vi "Rampe e compensazioni V F C.vi"(0 "Stato Rampe":refnum<vi>, 1 "Parametri inv freno":refnum<vi>, 2 "lingua":refnum<vi>, 3 "RPM PROVA":refnum<vi>, 5 "stato Parametri rampe e comp":refnum<vi>, 7 "COPPIA DI FRENATURA [Nm]":refnum<vi>, 9 "Tipo alimentatore DC":refnum<vi>, 11 "V F Prova":refnum<vi>, 12 "Tipo motore":refnum<vi>, 13 "Stato strumenti":refnum<vi>, 14 "Forza controllo vel":refnum<vi>) -> (15 "error out":errorcluster)   [LabVIEW 2019]
uses:
  Parametri rampe e comp.ctl
  <vilib>/ptbypt/NI_PtbyPt.lvlib
  PROVE/tensione simulata.vi
  cDAQ_PLC Folder/cDAQ/AO List.ctl
  cDAQ_PLC Folder/cDAQ/SET SINGLE AO.ctl
  Global_tutti_iDati.vi
  Global_scelta_banco.vi
  Global Modulo lingua.vi
  Global Coppia max tors.vi
panel:
  in  "exit":bool
  out "Stato Rampe":T1 {"Rampa C" scale=0.0..500.0; "Rampa V" scale=0.0..400.0; "Rampa Hz" scale=0.0..50.0}
  in  "precisione kw":dbl
  in  "RPM":dbl
  in  "RPM nom":dbl
  in  "P resa letta":dbl
  in  "P imp":dbl
  out "tensione stabilizzata":bool
  out "coppia stabilizzata":bool caption="Grandezza stabilizz?"
  out "Stato":string
  in  "set V (V)":dbl
  out "stato Parametri rampe e comp":T2={"Frequenza"={"Tempo rampa (s)"=0.0, "Tempo stabiliz (s)"=0.0}, "Tensione"={"Tempo rampa (s)"=0.0, "Tempo stabiliz rampa(s)"=0.0, "Compensaz attiva?"=TRUE, "Precisione"=1.0, "Delta compensazione max"=30.0, "Time attesa stabiliz comp (s)"=5.0}, "Coppia"={"Tempo rampa (s)"=0.0, "Tempo stabiliz rampa(s)"=0.0, "Compensaz attiva?"=TRUE, "Precisione"=1.0, "Delta compensazione max"=30.0, "Time attesa stabiliz comp (s)"=5.0}}
  in  "Parametri rampe e comp":T2={"Frequenza"={"Tempo rampa (s)"=0.0, "Tempo stabiliz (s)"=0.0}, "Tensione"={"Tempo rampa (s)"=0.0, "Tempo stabiliz rampa(s)"=0.0, "Compensaz attiva?"=TRUE, "Precisione"=1.0, "Delta compensazione max"=30.0, "Time attesa stabiliz comp (s)"=5.0}, "Coppia"={"Tempo rampa (s)"=0.0, "Tempo stabiliz rampa(s)"=0.0, "Compensaz attiva?"=TRUE, "Precisione"=1.0, "Delta compensazione max"=30.0, "Time attesa stabiliz comp (s)"=5.0}}
  out "Coppia letta":dbl
  out "Tensione letta":dbl
  out "fine rampa C":bool
  in  "set (C)":dbl
  out "OUT C":dbl
  out "fine rampa V":bool
  out "OUT V":dbl
  out "OUT HZ":dbl
  in  "set (Hz)":dbl
  out "fine rampa HZ":bool
  # "controlli per simulazione"
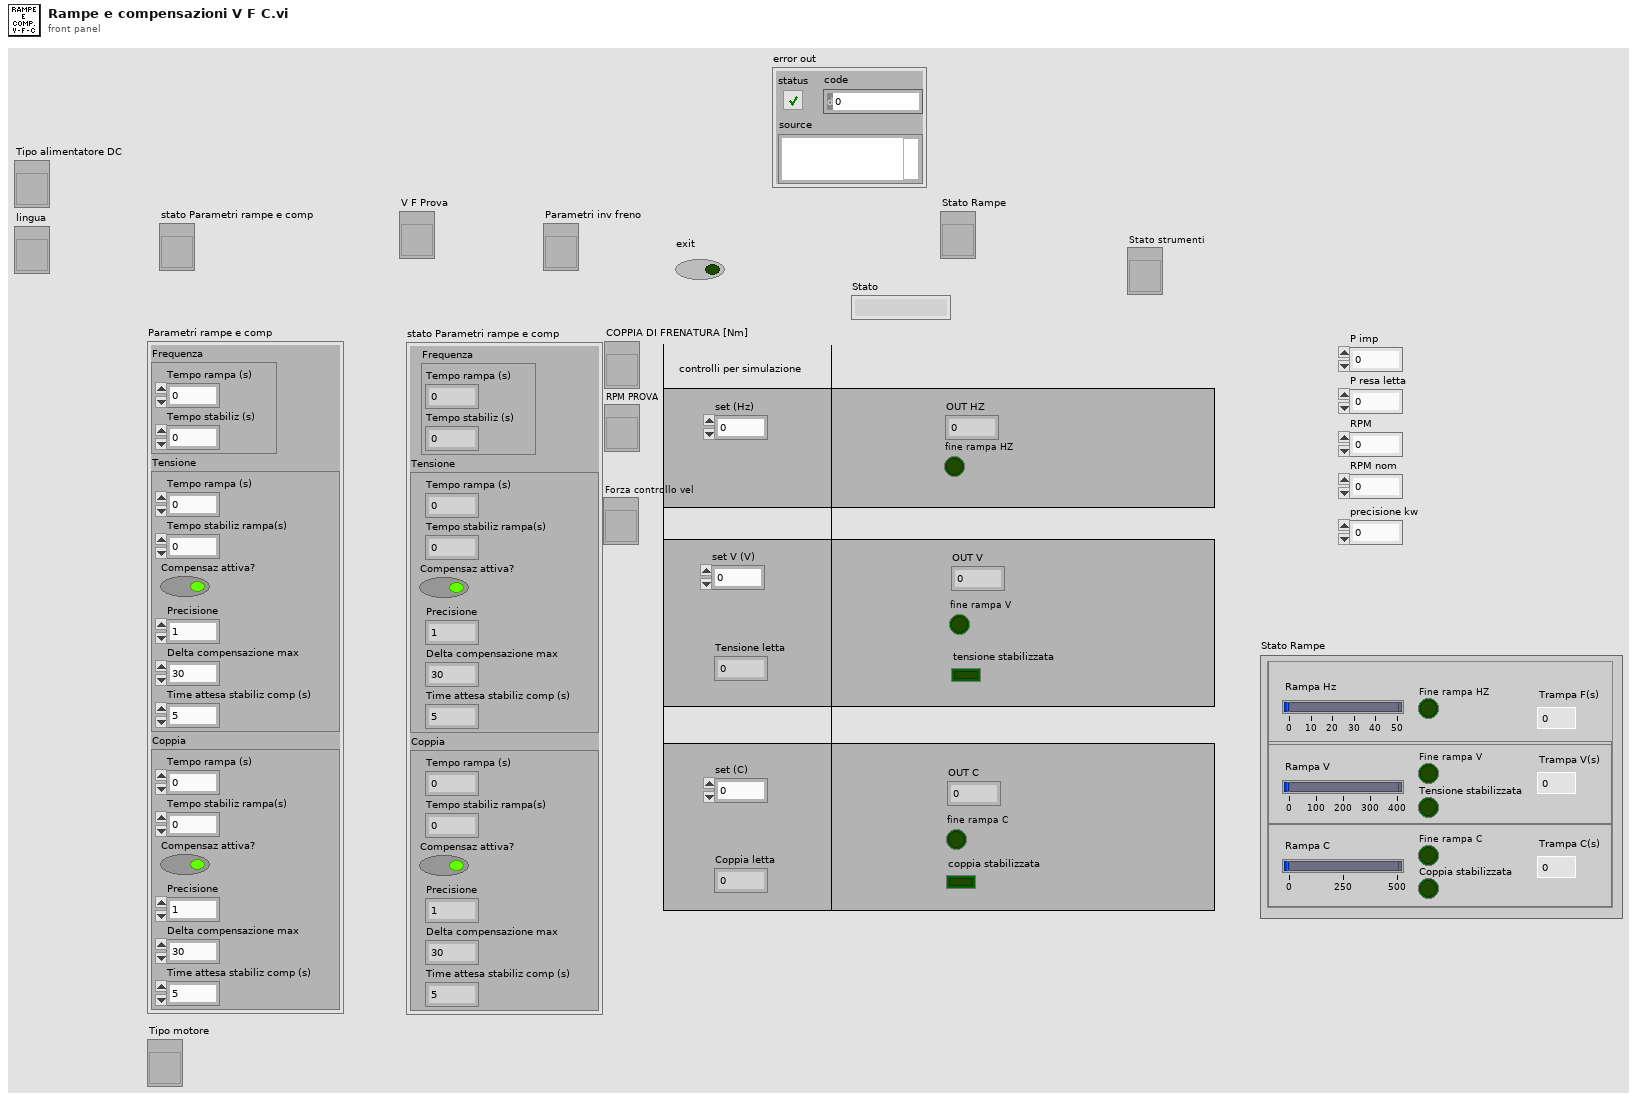
[diagram p1: front panel]
types:
  T1 = cluster{"Fine rampa HZ":bool, "Fine rampa V":bool, "Tensione stabilizzata":bool, "Fine rampa C":bool, "Coppia stabilizzata":bool, "Rampa Hz":dbl, "Rampa V":dbl, "Rampa C":dbl, "Trampa F(s)":dbl, "Trampa V(s)":dbl, "Trampa C(s)":dbl}
  T2 = typedef "Parametri rampe e comp.ctl" = cluster{"Frequenza":cluster{"Tempo rampa (s)":dbl, "Tempo stabiliz (s)":dbl}, "Tensione":cluster{"Tempo rampa (s)":dbl, "Tempo stabiliz rampa(s)":dbl, "Compensaz attiva?":bool, "Precisione":dbl, "Delta compensazione max":dbl, "Time attesa stabiliz comp (s)":dbl}, "Coppia":cluster{"Tempo rampa (s)":dbl, "Tempo stabiliz rampa(s)":dbl, "Compensaz attiva?":bool, "Precisione":dbl, "Delta compensazione max":dbl, "Time attesa stabiliz comp (s)":dbl}}
  T3 = cluster{"Message":string, "Message Data":variant}
  T4 = cluster{"name (unnamed)":string, "variant":variant}
  T5 = typedef "SET SINGLE AO.ctl" = cluster{"AO":T6, "Value":dbl}
  T6 = typedef "AO List.ctl" = enum16{"OFF: ALL AO", "Vout Variac", "Vout Freq", "Vout 3", "Vout 4", "Forza AO", "*V eccitazion", "*I eccitazione", "*Rif vel inv freno", "*Rif coppia inv freno", "Exit"}
  T7 = cluster{"WT330":bool, "CDAQ":bool, "RESIS. METER":bool, "PLC":bool, "AFE ENERGY":bool, "INV FRENO":bool, "RESISTOMAT":bool}
  T8 = typedef "Tutti_i_dati.ctl" = cluster{"Letture":T9, "Misure Wt330":cluster{"CANALE 1":cluster{"U":dbl, "I":dbl, "P":dbl, "S":dbl, "Q":dbl, "LAMB":dbl, "PHI":dbl, "FU":dbl, "FI":dbl, "NONE":dbl}, "CANALE 2":cluster{"U":dbl, "I":dbl, "P":dbl, "S":dbl, "Q":dbl, "LAMB":dbl, "PHI":dbl, "FU":dbl, "FI":dbl, "NONE":dbl}, "CANALE 3":cluster{"U":dbl, "I":dbl, "P":dbl, "S":dbl, "Q":dbl, "LAMB":dbl, "PHI":dbl, "FU":dbl, "FI":dbl, "NONE":dbl}, "SIGMA":cluster{"U":dbl, "I":dbl, "P":dbl, "S":dbl, "Q":dbl, "LAMB":dbl, "PHI":dbl, "FU":dbl, "FI":dbl, "NONE":dbl}}, "statoAO_PLC":T10, "statoDO_cDaq":T11, "StatoDO_PLC":T12, "statoAO_Cdaq":T13}
  T9 = typedef "LettureCDAQ_PLC.ctl" = cluster{"DI-logici":cluster{"Sistema OK":bool, "Inverter mot freno Run":bool, "Collaudo abilitato":bool, "Potenza trifase abilitata":bool, "Potenza monofase abilitata":bool, "Potenza DC abilitata":bool, "Potenza DC MP abilitata":bool, "Potenza DC abilitata no WT":bool, "Potenza DC MP abilitata no WT":bool, "Potenza Eccitazione abilitata":bool, "Start alimentazione AC":bool, "Start alimentazione DC":bool, "Start eccitazione DC":bool, "Controllo coppia abilitato":bool, "Senso rotazione motore freno":bool, "Teler ramo WT abilitato":bool, "Teler princ Resist abilitato":bool, "Teler corto fasi":bool, "Ramo 1 resistomat":bool, "Ramo 2 resistomat":bool, "Ramo 3 resistomat":bool, "Stop prova":bool, "Reset allarme":bool, "Rot bloccato (0= bloccato)":bool, "Scala torsiometro":bool}, "Termocoppie":cluster{"Tamb (°C)":dbl, "TC 2":dbl, "TC 3":dbl, "TC 4":dbl}, "AI cDAQ":cluster{"C[Nm] 1":dbl, "C[Nm] 2":dbl}, "Counters":cluster{"RPM 1":dbl, "RPM 2":dbl}, "Stato DI_Cdaq":cluster{"Motore monofase abil":bool, "Motore trifase abil":bool, "Uscita generale abil":bool, "2nd ch res meter abil":bool, "TA selezionati":bool, "Pulsante Start prova":bool, "Pulsante Stop prova":bool, "Pulsante Reset allarmi":bool, "Secondari TA aperti":bool, "Res meter abil":bool, "Scorta 1":bool, "Scorta 2":bool, "Scorta 3":bool, "Scorta 4":bool, "Scorta 5":bool, "Scorta 6":bool, "Scorta 7":bool, "Scorta 8":bool, "Scorta 9":bool, "Scorta 10":bool, "Scorta 11":bool, "Scorta 12":bool, "Scorta 13":bool, "Scorta 14":bool, "Scorta 15":bool, "Scorta 16":bool, "Scorta 17":bool, "Scorta 18":bool, "Scorta 19":bool, "Scorta 20":bool, "Scorta 21":bool, "Scorta 22":bool}, "Stato DI_PLC":cluster{"Diff Relay On":bool, "Em Stop Mod ok":bool, "Secur Bar Mod ok":bool, "Int PwPan Fan enab":bool, "Start Test P-b":bool, "Stop Test P-b":bool, "Reset Alarms P-b":bool, "Single-ph M enab":bool, "Three-ph M enab":bool, "Gen Output enab":bool, "Inv  11kW enab":bool, "Inv 3kW enab":bool, "AFE enab":bool, "P.S. Brushless M enab":bool, "Brush M started (scorta)":bool, "M Tested Sig enab":bool, "Br M 4kW Fan enab":bool, "Blocked Rot 1":bool, "Blocked Rot 2":bool, "Klixon Br Res 1":bool, "Klixon Br Res 2":bool, "Klixon Line Reac":bool, "Klixon S.L. Reac":bool, "Res Meter enab":bool, "2Ch Res Meter enab":bool, "Bypass Res Meter":bool, "TA selected":bool, "TA bypassed":bool, "Direct Line sel":bool, "Branch WT enab":bool, "Branch 1 Resist":bool, "Branch 2 Resist":bool, "Branch 3 Resist":bool, "Short Circ windings":bool, "Sec1 coil sel":bool, "Sec2 Coil sel":bool, "Inv 11kW ready":bool, "Inv 3kW ready":bool, "AFE ready":bool, "P.S. Direct Line enab":bool, "Scorta 1":bool, "Scorta 2":bool, "Scorta 3":bool, "Scorta 4":bool, "Scorta 5":bool, "Scorta 6":bool, "*Inv 11kW started":bool, "*Inv 3kW started":bool, "*AFE started":bool, "*Bench 300W":bool, "*Bench 3kW":bool}, "Letture res meter":cluster{"Res Ch1":dbl, "Res Ch2":dbl}, "Banco selez":cluster{"C[Nm]":dbl, "RPM":dbl}, "AI plc":cluster{"Allarmi_1":dbl, "Allarmi_2":dbl, "RPM inv 3kW":dbl, "RPM inv 11kW":dbl}, "Letture resistomat":cluster{"Res Ch1":dbl, "Res Ch2":dbl}}
  T10 = typedef "statoAO_plc.ctl" = cluster{"Rif vel freno":dbl, "Rif coppia freno":dbl, "Rif tens AFE":dbl, "Rif freq AFE":dbl}
  T11 = typedef "statoDO.ctl" = cluster{"Abilita motore monofase":bool, "Abilita motore trifase":bool, "Abilita uscita generale":bool, "Abilita res meter":bool, "Abilita 2nd canale res meter":bool, "Bypass res meter":bool, "Ctrl torsiometro 1":bool, "Scala torsiometro 1":bool, "Ctrl torsiometro 2":bool, "Scala torsiometro 2":bool, "Seleziona TA":bool, "Seleziona linea diretta":bool, "Seleziona spire TA":bool, "Bypass TA":bool, "Lampada Test in progress":bool, "Lampada allarme":bool, "Apri TA secondari":bool, "Scorta 1":bool, "Scorta 2":bool, "Scorta 3":bool, "Scorta 4":bool, "Scorta 5":bool, "Scorta 6":bool, "Scorta 7":bool, "Scorta 8":bool, "Scorta 9":bool, "Scorta 10":bool, "Scorta 11":bool, "Scorta 12":bool, "Scorta 13":bool, "Scorta 14":bool, "Scorta 15":bool}
  T12 = typedef "StatoDO_PLC.ctl" = cluster{"Enab Single-ph M":bool, "Enab Three-ph M":bool, "Enab Gen Output":bool, "Enab Electric Lock":bool, "Reset Diff Relay":bool, "Test in Progress Lamp":bool, "Alarm Lamp":bool, "Enab Inv 11kW":bool, "Start Inv 11kW":bool, "Scorta 1":bool, "Enab Inv 3kW":bool, "Start Inv 3kW":bool, "Enab AFE":bool, "Start AFE":bool, "Enab PS Brush M":bool, "Start Brush M (scorta)":bool, "Enab M Tested Sig":bool, "Enab Fan Brak M 4kW":bool, "Enab Res Meter":bool, "Enab 2Ch Res Meter":bool, "Bypass Res Meter":bool, "Select TA":bool, "Bypass TA":bool, "Select Direct Line":bool, "Enab Branch WT":bool, "Spire TA (scorta)":bool, "Ctrl Torq Meter 50Nm":bool, "Scale Torq Meter 50Nm ":bool, "Ctrl Torq Meter 5Nm":bool, "Scale Torq Meter 5Nm":bool, "Branch 1 resist":bool, "Branch 2 resist":bool, "Branch 3 resist":bool, "Short Circ Windings":bool, "Sel  Windings 300V":bool, "Sel  Windings 450V":bool, "P.S. Direct Line":bool, "Scorta 2":bool, "Scorta 3":bool, "Scorta 4":bool, "Scorta 5":bool, "Scorta 6":bool, "*Reset Allarmi":bool, "*Senso Rotaz freno":bool, "*Controllo Coppia":bool, "*Abilita freno":bool, "*Marcia freno":bool, "*Watch dog":bool, "*Bench 300W":bool, "*Bench 3kW":bool}
  T13 = typedef "StatoAO_cdaq.ctl" = cluster{"Vout variac":dbl, "AO 2":dbl, "AO 3":dbl, "AO 4":dbl}
  T14 = cluster{"Tempo rampa (s)":dbl, "Tempo stabiliz rampa(s)":dbl, "Compensaz attiva?":bool, "Precisione":dbl, "Delta compensazione max":dbl, "Time attesa stabiliz comp (s)":dbl}
  T15 = cluster{"Tempo rampa (s)":dbl, "Tempo stabiliz (s)":dbl}
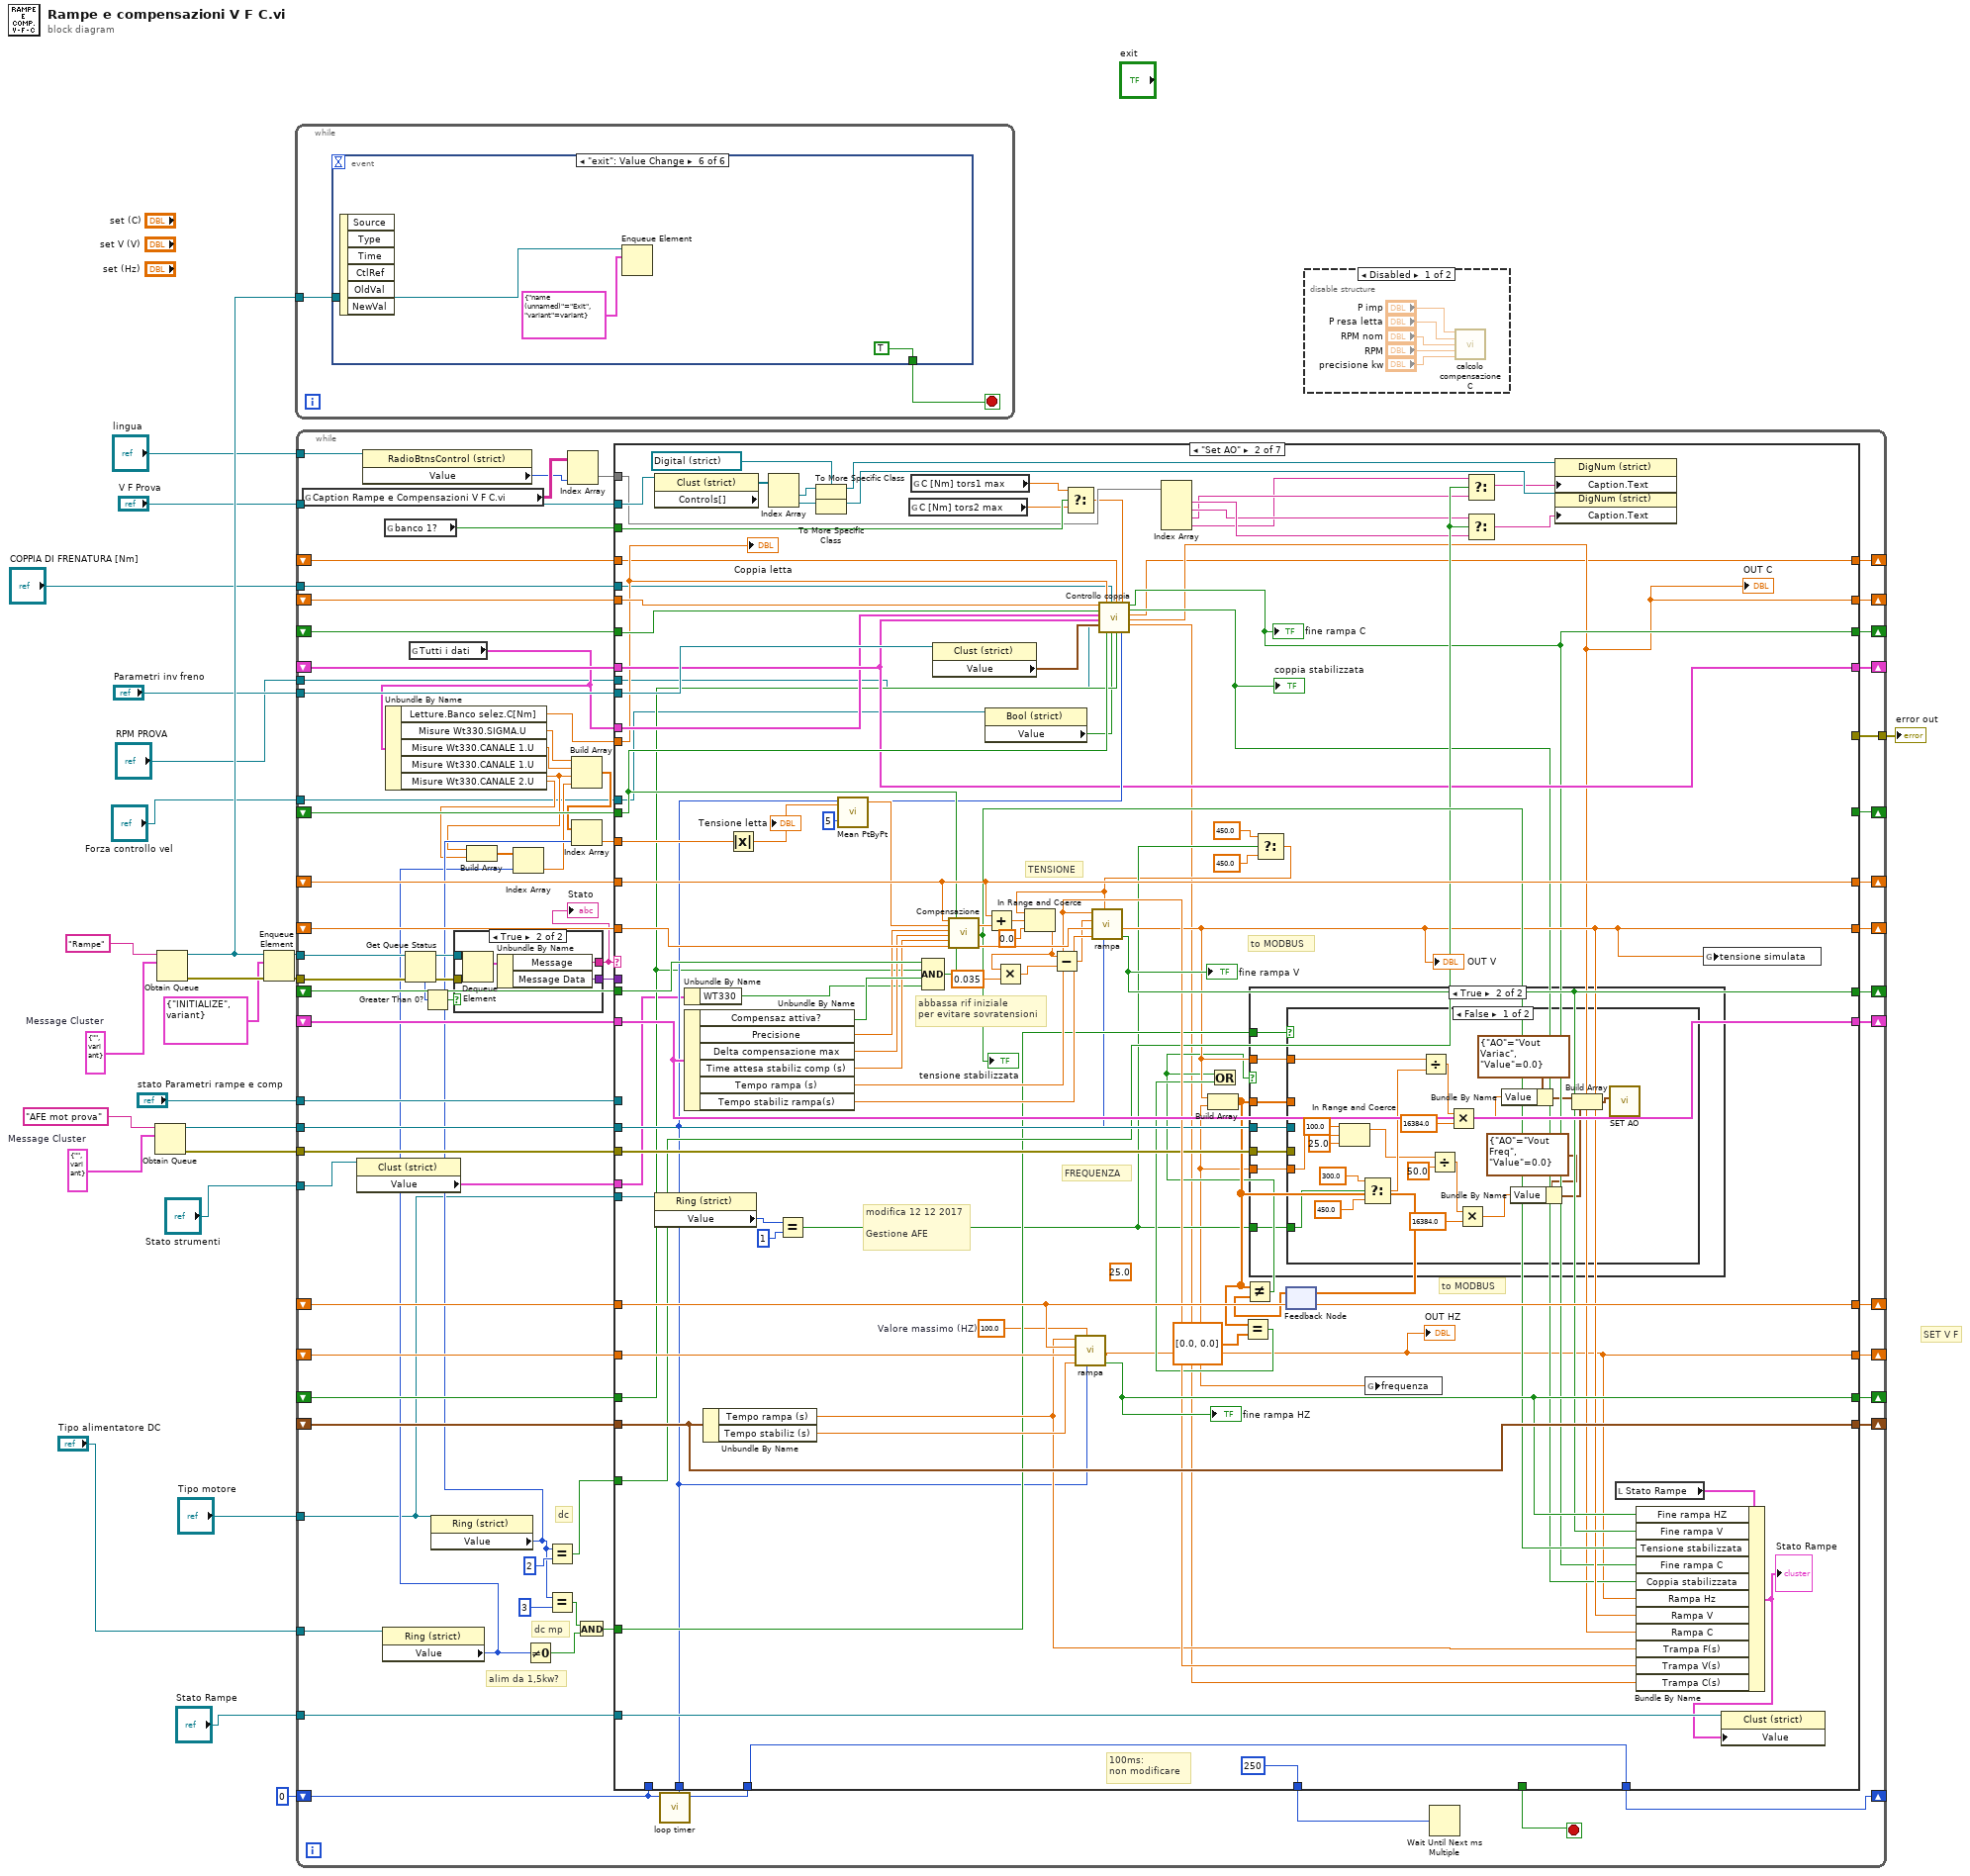
[diagram p0: block diagram]
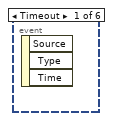
[diagram p3: hidden frame]
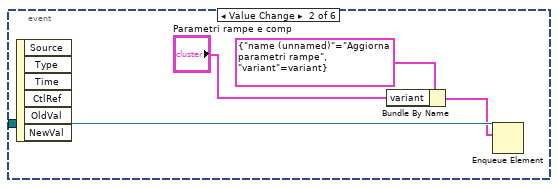
[diagram p4: hidden frame]
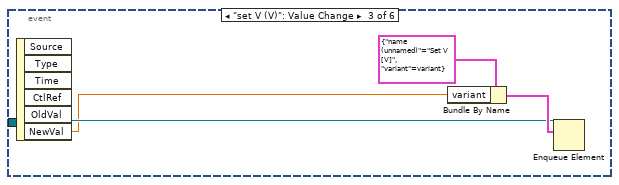
[diagram p5: hidden frame]
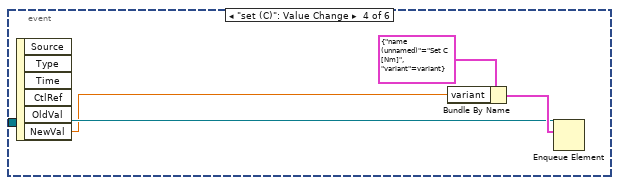
[diagram p6: hidden frame]
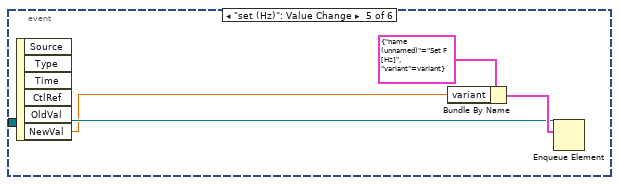
[diagram p7: hidden frame]
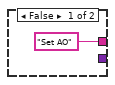
[diagram p8: hidden frame]
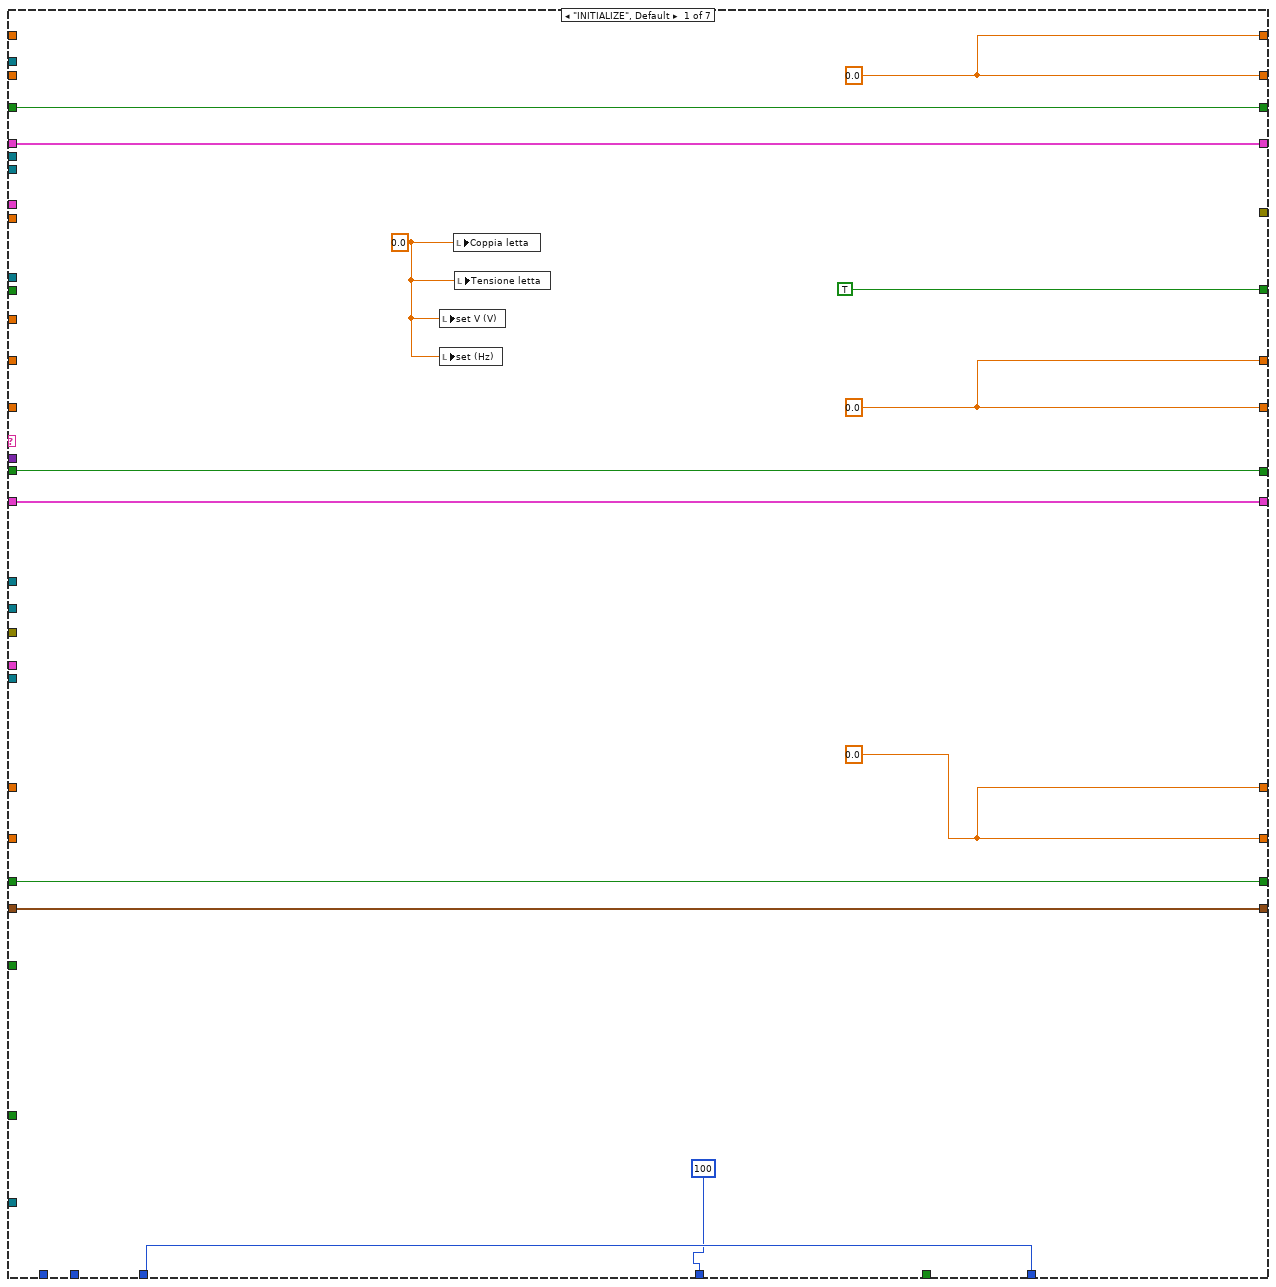
[diagram p9: hidden frame]
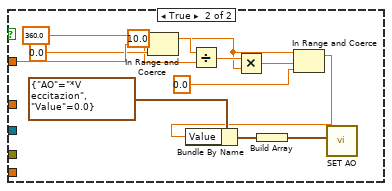
[diagram p11: hidden frame]
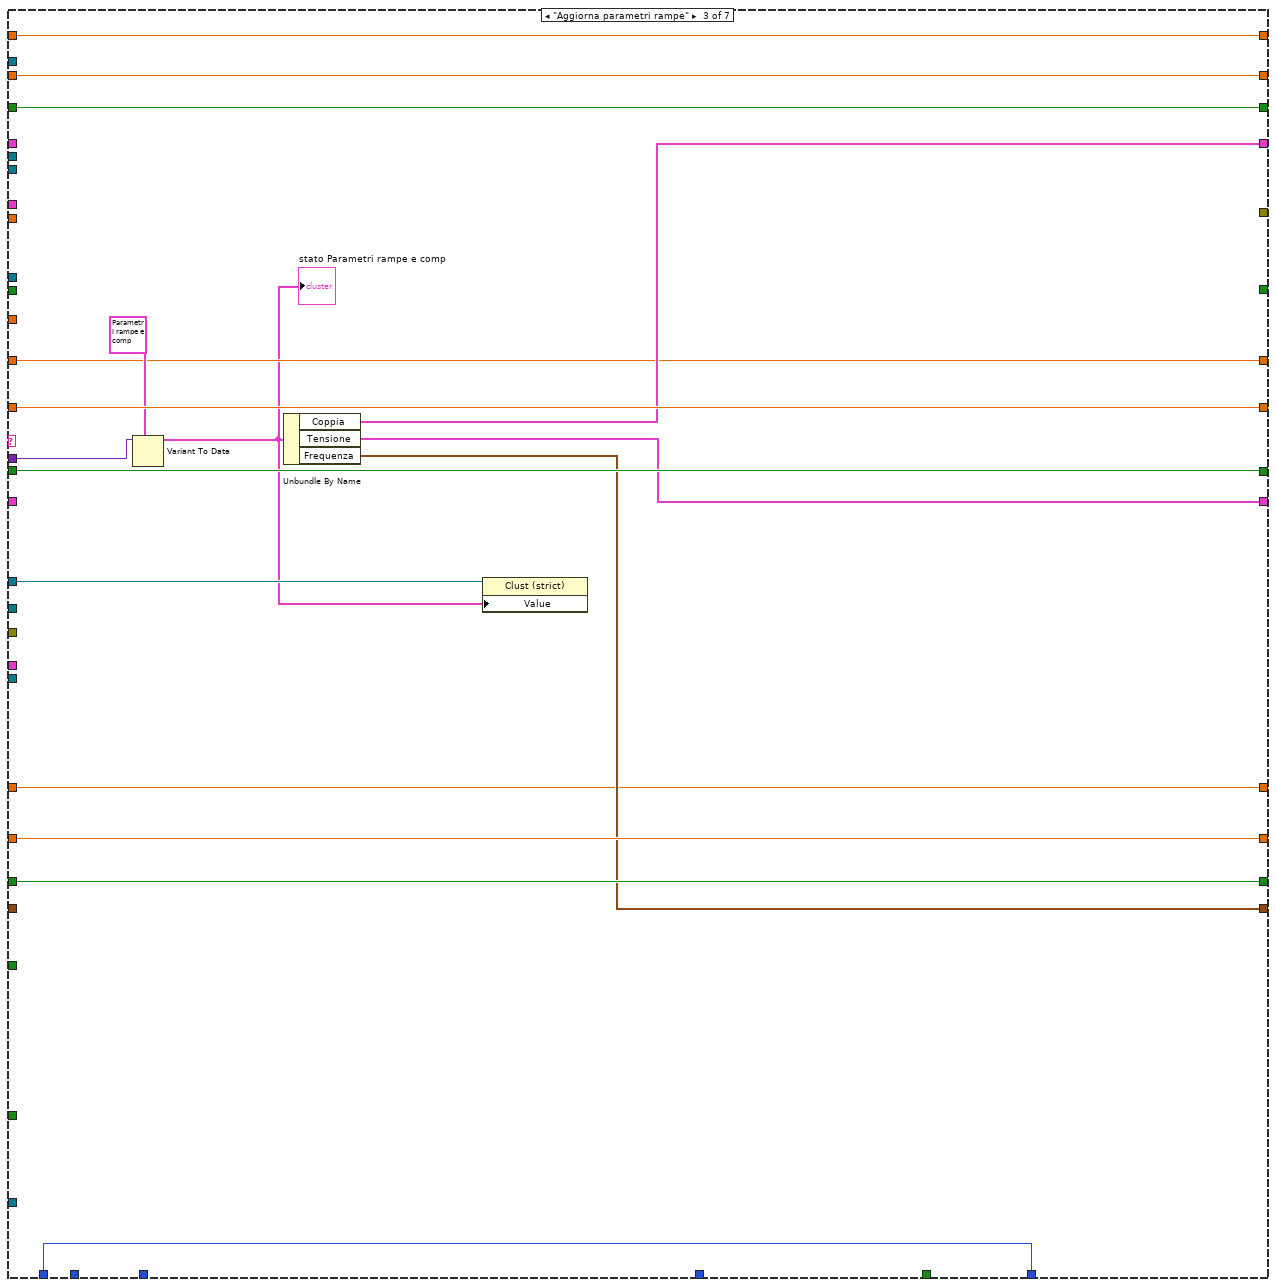
[diagram p12: hidden frame]
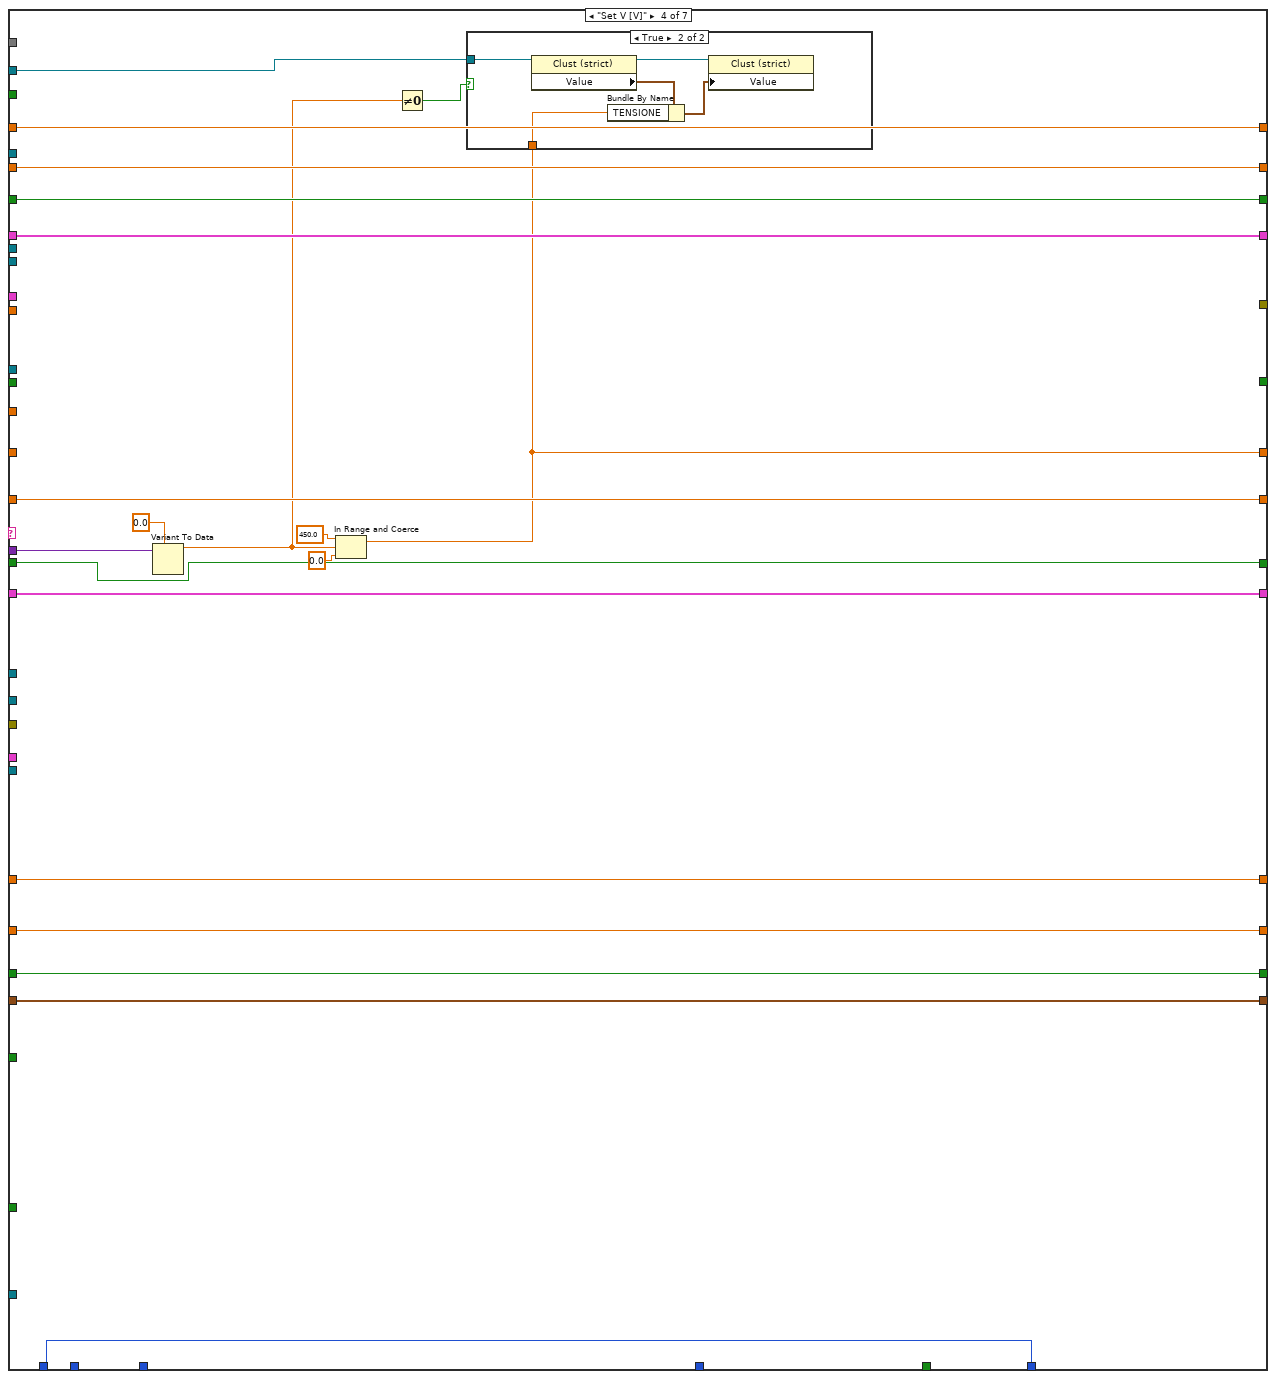
[diagram p13: hidden frame]
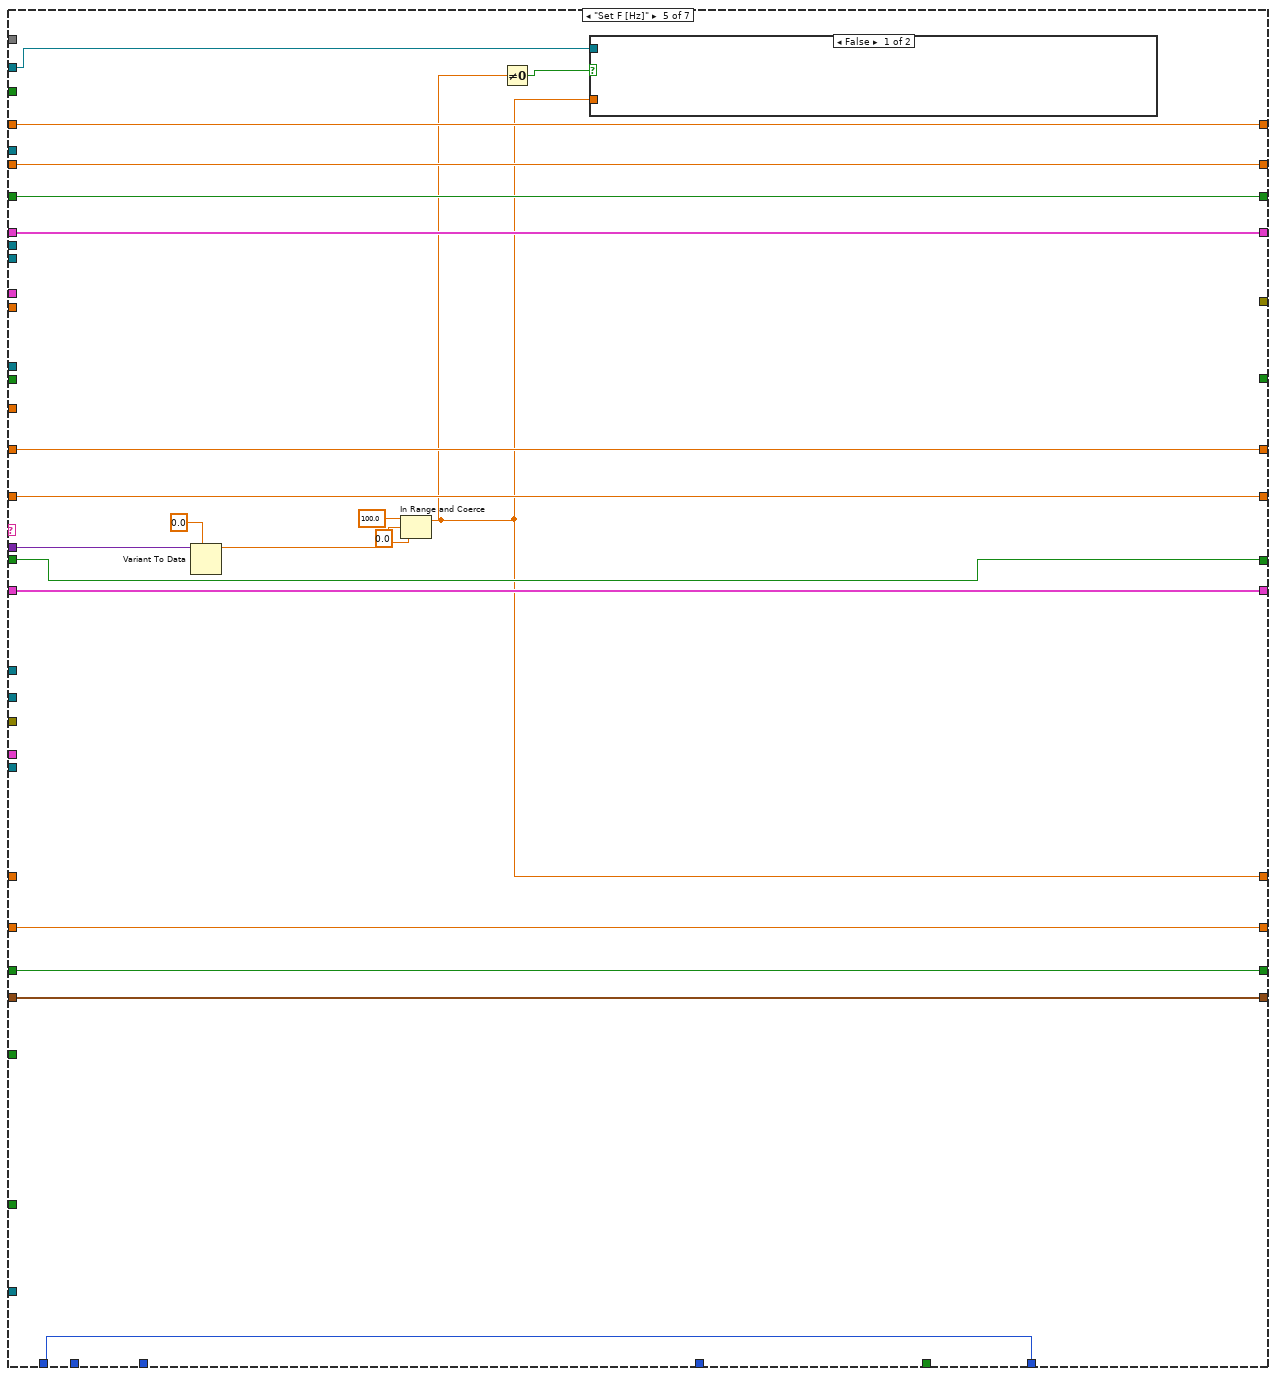
[diagram p15: hidden frame]
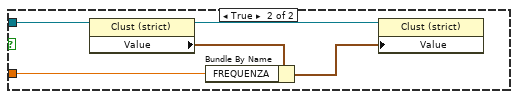
[diagram p16: hidden frame]
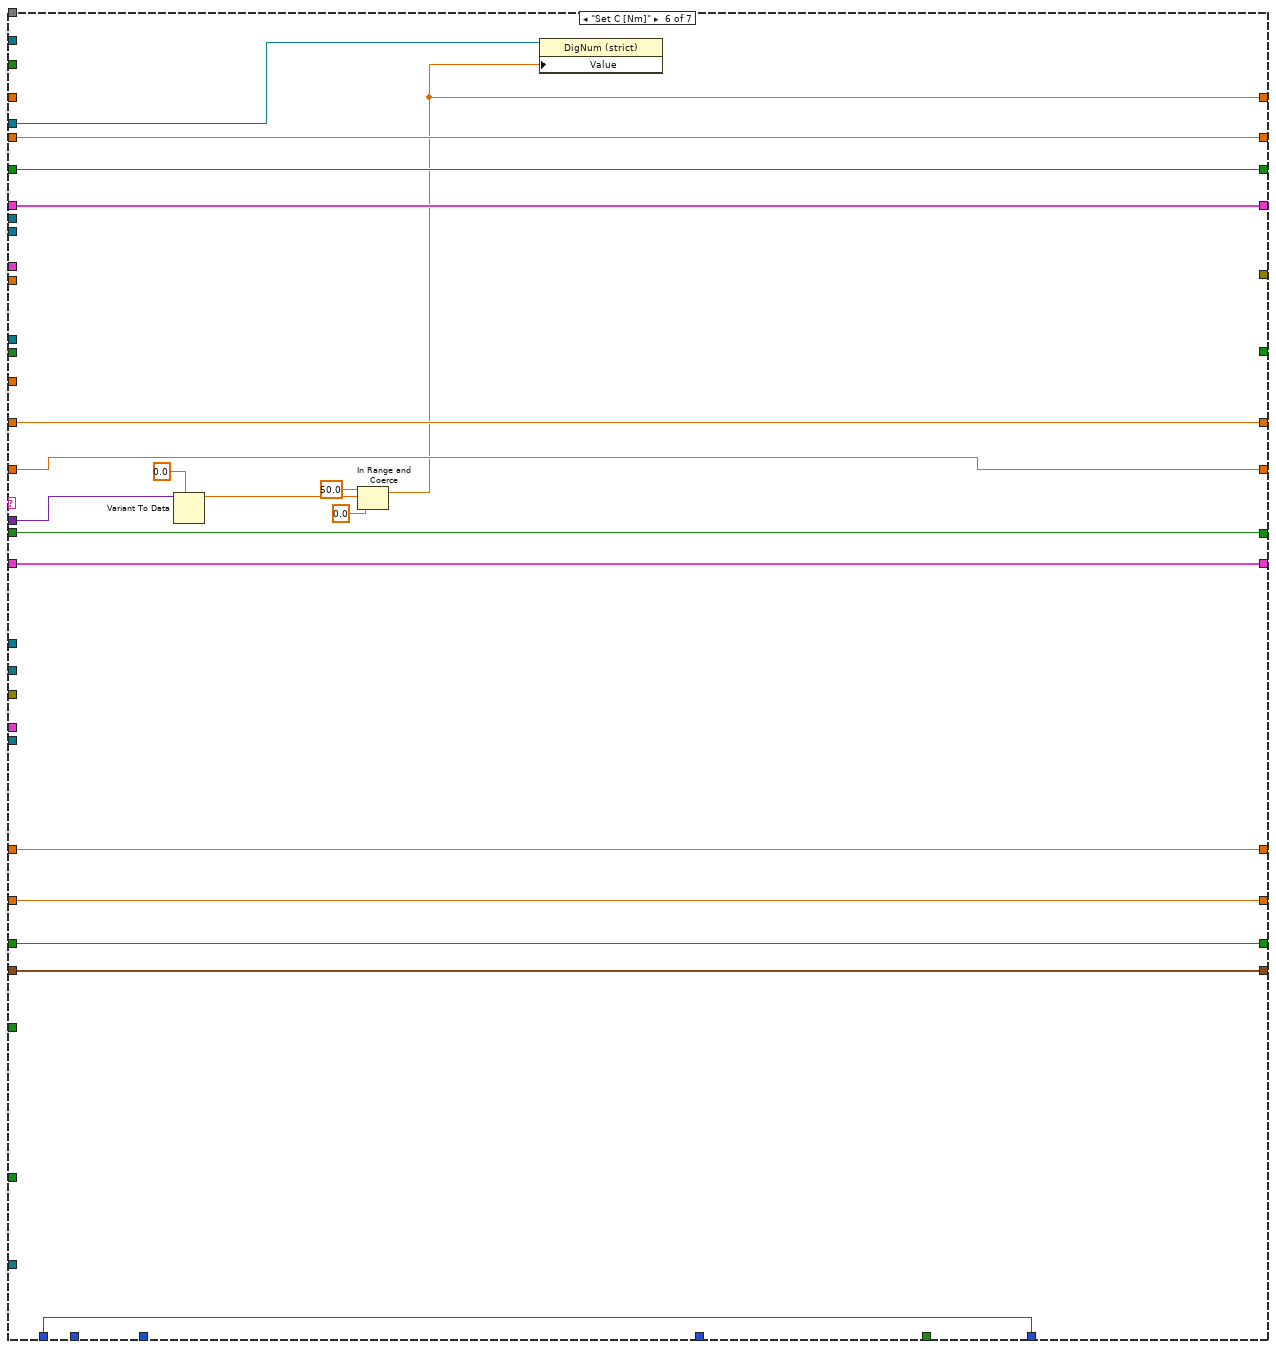
[diagram p17: hidden frame]
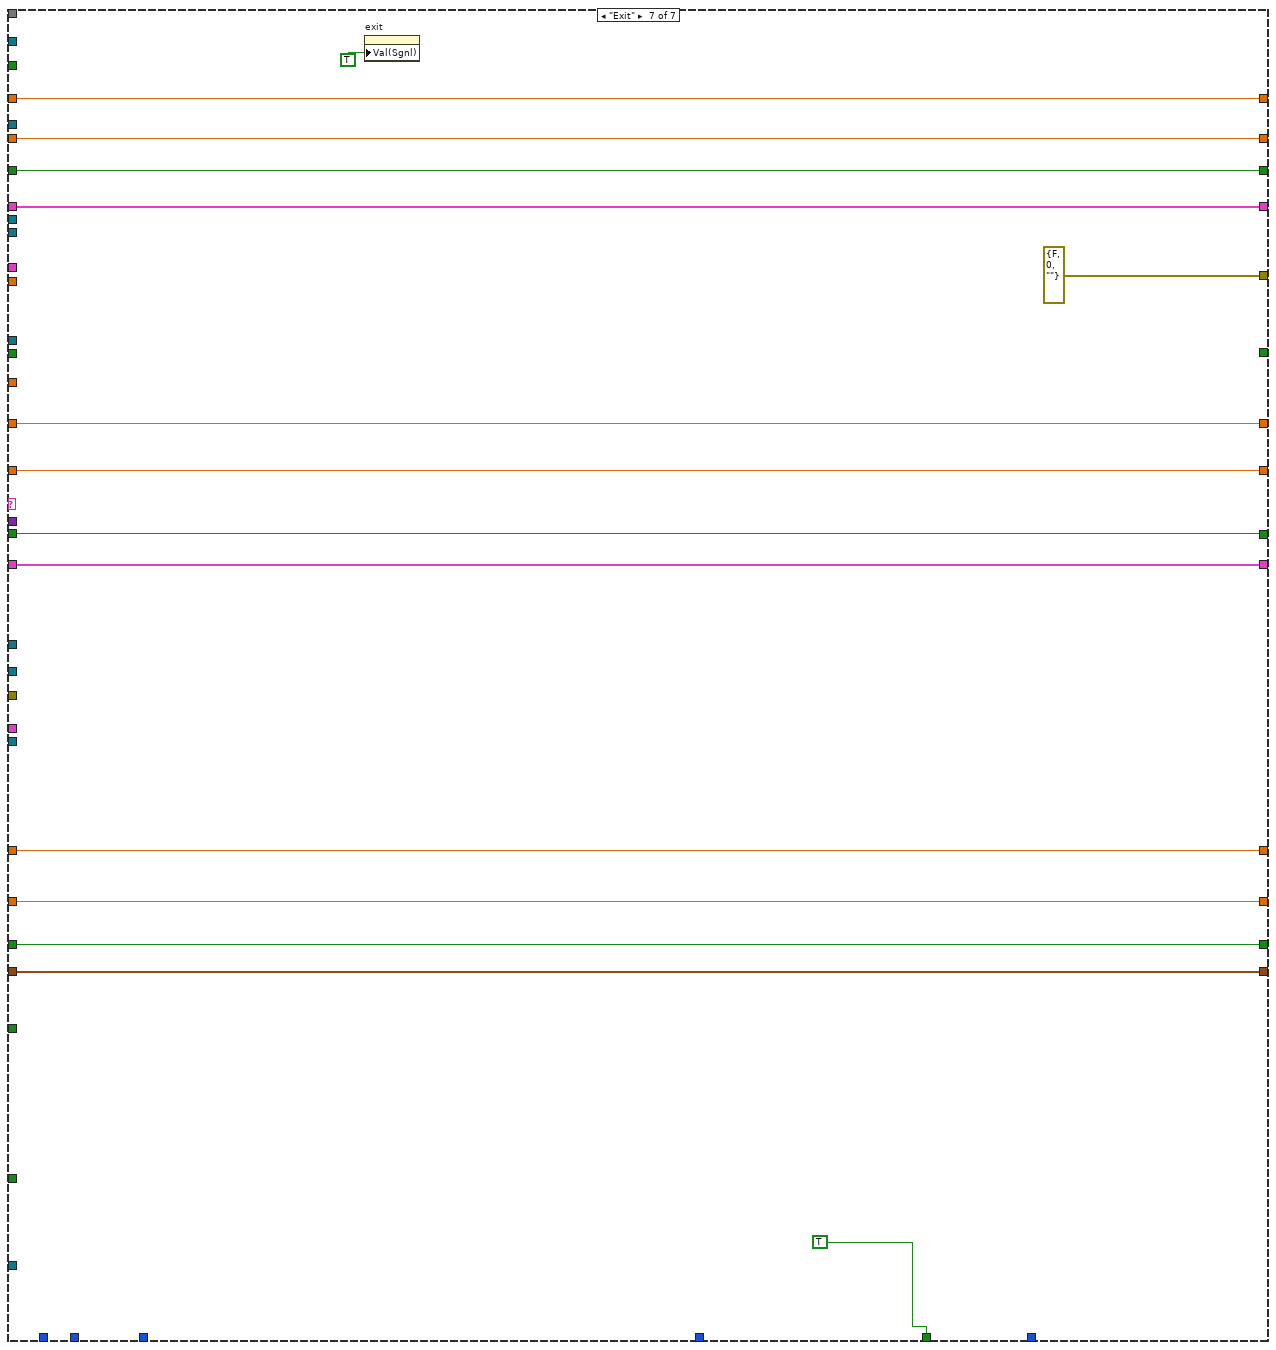
[diagram p18: hidden frame]
diagram:
  w13 = T3 {"Message"="", "Message Data"=variant}  # Message Cluster
  w17 = T3 {"Message"="", "Message Data"=variant}  # Message Cluster
  # "SET V F"
  n1 = Obtain Queue(name (unnamed)="AFE mot prova", element data type=w13) -> (queue out=w11:refnum<queue>, error out=w10:errorcluster)  [unwired: 3 in, 1 out]
  n2 = Obtain Queue(name (unnamed)="Rampe", element data type=w17) -> (queue out=w18:refnum<queue>, error out=w23:errorcluster)  [unwired: 3 in, 1 out]
  n3 = Enqueue Element(queue=w18, element=T4 {"name (unnamed)"="INITIALIZE", "variant"=variant}, error in (no error)=w23) -> (queue out=w21:refnum<queue>, error out=w22:errorcluster)  [unwired: 1 in, 1 out]
  n4 = while {
    tunnel: w18 -> [w26]
    stop <- w25 stop-if-true
    n5 = event shown="[5] \"exit\": Value Change" {
      selector: _ -> [_ _ _ _ _ _]
      dyn-events: _ -> [_ _ _ _ _ _]
      timeout: _ -> [_ _ _ _ _ _]
      tunnel: w26 -> [_ w30 w32 w36 w40 w43]
      tunnel: [_ _ _ _ _ TRUE] -> w25
      event Timeout {
        n6 = event-data() -> ()  [unwired: 1 in, 3 out]
      }
      event Value Change {
        n7 = event-data() -> ()  [unwired: 1 in, 6 out]
        n8 = Bundle By Name(cluster=T4 {"name (unnamed)"="Aggiorna parametri rampe", "variant"=variant}, "variant"="Parametri rampe e comp") -> (w29:T4)
        n9 = Enqueue Element(queue=w30, element=w29) -> ()  [unwired: 2 in, 3 out]
      }
      event "set V (V)": Value Change {
        n10 = event-data() -> ("NewVal"=w31:dbl)  [unwired: 1 in, 5 out]
        n11 = Bundle By Name(cluster=T4 {"name (unnamed)"="Set V [V]", "variant"=variant}, "variant"=w31) -> (w34:T4)
        n12 = Enqueue Element(queue=w32, element=w34) -> ()  [unwired: 2 in, 3 out]
      }
      event "set (C)": Value Change {
        n13 = event-data() -> ("NewVal"=w35:dbl)  [unwired: 1 in, 5 out]
        n14 = Bundle By Name(cluster=T4 {"name (unnamed)"="Set C [Nm]", "variant"=variant}, "variant"=w35) -> (w38:T4)
        n15 = Enqueue Element(queue=w36, element=w38) -> ()  [unwired: 2 in, 3 out]
      }
      event "set (Hz)": Value Change {
        n16 = event-data() -> ("NewVal"=w39:dbl)  [unwired: 1 in, 5 out]
        n17 = Bundle By Name(cluster=T4 {"name (unnamed)"="Set F [Hz]", "variant"=variant}, "variant"=w39) -> (w42:T4)
        n18 = Enqueue Element(queue=w40, element=w42) -> ()  [unwired: 2 in, 3 out]
      }
      event "exit": Value Change {
        n19 = event-data() -> ()  [unwired: 1 in, 6 out]
        n20 = Enqueue Element(queue=w43, element=T4 {"name (unnamed)"="Exit", "variant"=variant}) -> ()  [unwired: 2 in, 3 out]
      }
    }
  }
  n21 = while {
    shift-right: [w77] -> _
    shift-left: u32 0 ("millisecond timer OUT") -> [w76]
    shift-right: [w121] -> _
    shift-left: _ -> [w122]
    shift-right: [w120] -> _
    shift-left: _ -> [w112]
    shift-right: [w118] -> _
    shift-left: _ -> [w119]
    shift-right: [w116] -> _
    shift-left: _ -> [w113]
    shift-right: [w115] -> _
    shift-left: _ -> [w114]
    shift-right: [w111] -> _
    shift-left: _ -> [w110]
    tunnel: w21 -> [w108]
    tunnel: w22 -> [w109]
    shift-right: [w101] -> _
    shift-left: _ -> [w98]
    shift-right: [w100] -> _
    shift-left: _ -> [w96]
    shift-right: [w99] -> _
    shift-left: _ -> [w97]
    shift-right: [w95] -> _
    shift-left: _ -> [w94]
    shift-right: [w93] -> _
    shift-left: _ -> [w90]
    shift-right: [w92] -> _
    shift-left: _ -> [w91]
    shift-right: [w89] -> _
    shift-left: _ -> [w88]
    tunnel: "Stato Rampe" -> [w87]
    tunnel: "stato Parametri rampe e comp" -> [w86]
    tunnel: "V F Prova" -> [w85]
    tunnel: w11 -> [w83]
    tunnel: w10 -> [w82]
    tunnel: "Tipo motore" -> [w56]
    tunnel: "Parametri inv freno" -> [w75]
    tunnel: [w73] -> w7
    tunnel: "Tipo alimentatore DC" -> [w70]
    tunnel: "lingua" -> [w54]
    tunnel: "COPPIA DI FRENATURA [Nm]" -> [w50]
    tunnel: "Stato strumenti" -> [w49]
    tunnel: "RPM PROVA" -> [w47]
    tunnel: "Forza controllo vel" -> [w46]
    stop <- w74 stop-if-true
    # "alim da 1,5kw?"
    # "dc mp"
    # "dc"
    n22 = global read "Global Modulo lingua.vi" "Caption Rampe e Compensazioni V F C.vi"() -> (w53:string[][])
    n23 = property class="Clust (strict)"(reference=w49) -> ("Value"=w48:T7)  [unwired: 1 in, 2 out]
    n24 = property class="RadioBtnsControl (strict)"(reference=w54) -> ("Value"=w52:enum32{"Italiano", "English"})  [unwired: 1 in, 2 out]
    n25 = property class="Ring (strict)"(reference=w70) -> ("Value"=w58:u16)  [unwired: 1 in, 2 out]
    n26 = global read "Global_scelta_banco.vi" "banco 1?"() -> (w55:bool)
    n27 = Get Queue Status(queue=w108, error in (no error)=w109) -> (queue out=w104:refnum<queue>, error out=w105:errorcluster, # elements in queue=w107:i32)  [unwired: 1 in, 5 out]
    n28 = global read "Global_tutti_iDati.vi" "Tutti i dati"() -> (w57:T8)
    n29 = Unbundle By Name(w57) -> ("Letture.Banco selez.C[Nm]"=w84:dbl, "Misure Wt330.SIGMA.U"=w67:dbl, "Misure Wt330.CANALE 1.U"=w66:dbl, "Misure Wt330.CANALE 1.U"=w62:dbl, "Misure Wt330.CANALE 2.U"=w61:dbl)
    n30 = Greater Than 0?(x=w107) -> (x > 0?=w106:bool)
    n31 = property class="Ring (strict)"(reference=w56) -> ("Value"=w64:u16)  [unwired: 1 in, 2 out]
    n32 = case shown="True" w106 {
      tunnel: w105 -> [_ w128]
      tunnel: w104 -> [_ w127]
      tunnel: ["Set AO" ("Stato") w125] -> w103
      tunnel: [_ w124] -> w102
      frame False {
      }
      frame True {
        n33 = Dequeue Element(queue=w127, error in (no error)=w128) -> (element=w126:T3)  [unwired: 1 in, 3 out]
        n34 = Unbundle By Name(w126) -> ("Message"=w125:string, "Message Data"=w124:variant)
      }
    }
    "Stato" <- w103
    n35 = Build Array(w62, w61) -> (w60:dbl[])
    n36 = Index Array(array=w60, index=w58) -> (element=w59:dbl)
    n37 = Not Equal To 0?(x=w58) -> (x != 0?=w69:bool)
    n38 = Equal?(x=w64, y=u16 2) -> (x = y?=w80:bool)
    n39 = Equal?(x=w64, y=u16 3) -> (x = y?=w71:bool)
    n40 = Index Array(array=w53, index (col)=w52) -> (element=w51:string[])  [unwired: 1 in]
    n41 = Build Array(w67, w66, w62, w59) -> (w65:dbl[])
    n42 = Index Array(array=w65, index=w64) -> (element=w63:dbl)
    n43 = And(x=w71, y=w69) -> (x .and. y?=w68:bool)
    n44 = call <userlib>:"loop timer.vi"("millisecond timer IN"=w76) -> ("millisecond timer OUT"=w78:u32, "LOOP TIME (ms)"=w117:u32)  [unwired: 9 in]
    n45 = case shown="\"Set AO\"" w103 {
      tunnel: w122 -> [_ w236 w291 w307 w328 w355 w377]
      tunnel: [w133 w148 w291 w307 w328 w355 w377] -> w121
      tunnel: [w134 w188 w292 w303 w334 w358 w376] -> w120
      tunnel: w119 -> [_ w170 w293 w304 w329 w352 w375]
      tunnel: [w135 w162 w293 w304 w329 w352 w375] -> w118
      tunnel: w117 -> [_ w167 _ _ _ _ _]
      tunnel: [w136 w216 w289 w306 w331 w354 w374] -> w116
      tunnel: [w137 w215 w290 w309 w333 w357 w373] -> w115
      tunnel: w114 -> [w137 w235 w290 w309 w333 w357 w373]
      tunnel: w113 -> [w136 w152 w289 w306 w331 w354 w374]
      tunnel: w112 -> [_ w230 w292 w303 w334 w358 w376]
      tunnel: [w138 w164 w288 w311 w336 w360 w372] -> w111
      tunnel: w110 -> [w138 w166 w288 w311 w336 w360 w372]
      tunnel: w102 -> [_ _ w287 w313 w337 w361 _]
      tunnel: [w141 w165 w285 w310 w335 w359 w371] -> w101
      tunnel: [w140 w223 w284 w308 w332 w356 w370] -> w100
      tunnel: [w139 w222 w283 w305 w330 w353 w369] -> w99
      tunnel: w98 -> [w141 w165 _ w310 w335 w359 w371]
      tunnel: w96 -> [w140 w223 _ w308 w332 w356 w370]
      tunnel: w97 -> [w139 w222 _ w305 w330 w353 w369]
      tunnel: [w134 w221 w282 w297 w327 w351 w368] -> w95
      tunnel: w94 -> [_ w221 w282 _ w327 w351 w368]
      tunnel: [w133 w220 w281 w302 w320 w350 w367] -> w93
      tunnel: [w135 w146 w280 w301 w326 w344 w366] -> w92
      tunnel: w91 -> [_ w147 w280 w301 w326 _ w366]
      tunnel: w90 -> [_ w220 w281 w302 _ w350 w367]
      tunnel: [TRUE ("fine rampa") _ _ _ _ _ _] -> w89
      tunnel: w88 -> [_ w169 _ _ _ _ _]
      tunnel: w87 -> [_ w213 _ _ _ _ _]
      tunnel: w86 -> [_ _ w279 _ _ _ _]
      tunnel: w85 -> [_ w207 _ w300 w325 _ _]
      tunnel: w84 -> [_ w157 _ _ _ _ _]
      tunnel: w83 -> [_ w209 _ _ _ _ _]
      tunnel: w82 -> [_ w208 _ _ _ _ _]
      tunnel: w80 -> [_ w198 _ _ _ _ _]
      tunnel: w57 -> [_ w160 _ _ _ _ _]
      tunnel: [u32 100 ("millisecond multiple") u32 250 ("millisecond multiple") _ _ _ _ _] -> w79
      tunnel: w78 -> [w130 w196 _ _ _ _ _]
      tunnel: [w130 w196 w277 w296 w321 w346 _] -> w77
      tunnel: w76 -> [_ _ w277 w296 w321 w346 _]
      tunnel: w75 -> [_ w195 _ _ _ _ _]
      tunnel: [_ _ _ _ _ _ TRUE ("stop")] -> w74
      tunnel: [_ _ _ _ _ _ errorcluster {"status"=FALSE, "code"=0, "source"=""} ("error out")] -> w73
      tunnel: w68 -> [_ w189 _ _ _ _ _]
      tunnel: w63 -> [_ w187 _ _ _ _ _]
      tunnel: w55 -> [_ w185 _ _ _ _ _]
      tunnel: w56 -> [_ w184 _ _ _ _ _]
      tunnel: w51 -> [_ w180 _ _ _ _ _]
      tunnel: w50 -> [_ w142 _ _ _ w345 _]
      tunnel: w48 -> [_ w151 _ _ _ _ _]
      tunnel: w47 -> [_ w145 _ _ _ _ _]
      tunnel: w46 -> [_ w144 _ _ _ _ _]
      frame "INITIALIZE", Default {
        w131 = 0.0 ("Coppia reale letta")
        w135 = 0.0 ("OUT")
        w134 = 0.0 ("OUT")
        w133 = 0.0 ("OUT")
        n46 = local write "set V (V)"(w131) -> ()
        n47 = local write "set (Hz)"(w131) -> ()
        n48 = local write "Coppia letta"(w131) -> ()
        n49 = local write "Tensione letta"(w131) -> ()
      }
      frame "Set AO" {
        (unwired) 25.0 ("lower limit")
        w203 = refnum<vi> refnum ("Coppia letta")
        w149 = 100.0  # Valore massimo (HZ)
        # "abbassa rif iniziale\nper evitare sovratensioni"
        # "modifica 12 12 2017\n\nGestione AFE"
        # "100ms:\nnon modificare"
        # "to MODBUS"
        # "to MODBUS"
        # "TENSIONE"
        # "FREQUENZA"
        n50 = property class="Clust (strict)"(reference=w207) -> ("Controls[]"=w206:refnum<vi>[])  [unwired: 1 in, 2 out]
        n51 = property class="Ring (strict)"(reference=w184) -> ("Value"=w183:u16)  [unwired: 1 in, 2 out]
        n52 = Unbundle By Name(w151) -> ("WT330"=w150:bool)
        n53 = Unbundle By Name(w223) -> ("Compensaz attiva?"=w228:bool, "Precisione"=w225:dbl, "Delta compensazione max"=w226:dbl, "Time attesa stabiliz comp (s)"=w227:dbl, "Tempo rampa (s)"=w211:dbl, "Tempo stabiliz rampa(s)"=w229:dbl)
        n54 = Unbundle By Name(w222) -> ("Tempo rampa (s)"=w210:dbl, "Tempo stabiliz (s)"=w224:dbl)
        n55 = Absolute Value(x=w187) -> (abs(x)=w190:dbl)
        "Tensione letta" <- w190
        n56 = Index Array(array=w206) -> (element #1=w205:refnum<vi>, element #2=w204:refnum<vi>)  [unwired: 2 in]
        n57 = Equal?(x=w183, y=u16 1) -> (x = y?=w181:bool)
        n58 = To More Specific Class(target class=w203, reference=w205) -> (specific class reference=w202:refnum<vi>)  [unwired: 1 in, 1 out]
        n59 = To More Specific Class(target class=w203, reference=w204) -> (specific class reference=w201:refnum<vi>)  [unwired: 1 in, 1 out]
        n60 = call <vilib>:"Mean PtByPt.vi"("x"=w190, "sample length"=5) -> ("mean"=w218:dbl)  [unwired: 2 in, 1 out]
        n61 = global read "Global Coppia max tors.vi" "C [Nm] tors2 max"() -> (w174:dbl)
        n62 = global read "Global Coppia max tors.vi" "C [Nm] tors1 max"() -> (w175:dbl)
        n63 = Compound Arithmetic op=AND(w235, w152, w228, w150) -> (w233:bool)
        n64 = property class="Clust (strict)"(reference=w195) -> ("Value"=w168:cluster{"Vel max(RPM)":dbl, "Cmax (nm)":dbl})  [unwired: 1 in, 2 out]
        n65 = call "Compensazione.vi"("Grandezza target"=w221, "Grandezza reale letta"=w218, "Precisione"=w225, "Delta compensazione max"=w226, "Time attesa stabilizzazione (s)"=w227, "Grandezza attuale in"=w230, "Reset comp?"=w169, "Compensazione abilitata"=w233) -> ("compensazione"=w232:dbl, "Grandezza stabilizz?"=w214:bool, "Grandezza attuale out"=w231:dbl)  [unwired: 9 in]
        "tensione stabilizzata" <- w214
        n66 = property class="Bool (strict)"(reference=w144) -> ("Value"=w143:bool)  [unwired: 1 in, 2 out]
        n67 = Add(x=w221, y=w232) -> (x+y=w234:dbl)
        n68 = Select(t=w175, s=w185, f=w174) -> (s? t:f=w171:dbl)
        n69 = call "rampa.vi"("tempo ciclo (ms)"=w167, "Valore massimo"=w149, "Tempo di stabilizzazione (s)"=w224, "reale"=w236, "set"=w220, "tempo rampa (s)"=w210) -> ("fine rampa"=w216:bool, "OUT"=w148:dbl)  [unwired: 4 in]
        "fine rampa HZ" <- w216
        "OUT HZ" <- w148
        n70 = call "Controllo coppia.vi"("C attuale"=w170, "fine rampa C in"=w166, "Tutti i dati"=w160, "Coppia"=w165, "Cmax RPMmax\n inverter"=w168, "RPM PROVA"=w145, "Coppia letta tors"=w157, "Reset comp"=w169, "COPPIA DI FRENATURA [Nm]"=w142, "Forza controllo vel"=w143, "Set C"=w147, "Fine rampa F"=w152, "Cmax"=w171, "LOOP TIME (ms)"=w167) -> ("fine rampa C out"=w164:bool, "C stabile"=w163:bool, "Set C out"=w146:dbl, "Out C"=w162:dbl, "Tempo rampa (s)"=w161:dbl)  [unwired: 1 in]
        "OUT C" <- w162
        "fine rampa C" <- w164
        "coppia stabilizzata" <- w163
        n71 = Index Array(array=w180) -> (element #1=w179:string, element #2=w178:string, element #3=w177:string, element #4=w176:string)  [unwired: 4 in]
        n72 = Select(t=450.0 ("y"), s=w181, f=450.0) -> (s? t:f=w172:dbl)
        n73 = In Range and Coerce(upper limit=w172, x=w234, lower limit=0.0) -> (coerced(x)=w155:dbl)  [unwired: 1 out]
        n74 = Multiply(x=w155, y=0.035) -> (x*y=w154:dbl)
        n75 = Subtract(x=w155, y=w154) -> (x-y=w156:dbl)
        n76 = call "rampa.vi"("tempo ciclo (ms)"=w167, "Valore massimo"=w172, "Tempo di stabilizzazione (s)"=w229, "reale"=w231, "set"=w156, "tempo rampa (s)"=w211) -> ("fine rampa"=w215:bool, "OUT"=w188:dbl)  [unwired: 4 in]
        "fine rampa V" <- w215
        "OUT V" <- w188
        n77 = Build Array(w188, w148) -> (w193:dbl[])
        n78 = Equal?(x=w193, y=dbl[] [0.0, 0.0]) -> (x = y?=w191:bool)
        n79 = feedback-in #1(w193) -> ()
        n80 = feedback #1() -> (w194:dbl[])  [unwired: 1 in]
        n81 = Not Equal?(x=w193, y=w194) -> (x != y?=w186:bool)
        n82 = Or(x=w186, y=w191) -> ()  [unwired: 1 out]
        n83 = case shown="True" w186 {
          tunnel: w209 -> [_ w243]
          tunnel: w208 -> [_ w242]
          tunnel: w193 -> [_ w241]
          tunnel: w189 -> [_ w240]
          tunnel: w188 -> [_ w239]
          tunnel: w148 -> [_ w238]
          tunnel: w181 -> [_ w237]
          frame False {
          }
          frame True {
            n84 = case shown="False" w240 {
              tunnel: w243 -> [_ _]
              tunnel: w242 -> [_ _]
              tunnel: w241 -> [_ _]
              tunnel: w239 -> [w258 w271]
              tunnel: w238 -> [w245 _]
              tunnel: w237 -> [w251 _]
              frame False {
                n85 = In Range and Coerce(upper limit=100.0, x=w245, lower limit=25.0) -> (coerced(x)=w244:dbl)  [unwired: 1 out]
                n86 = Select(t=300.0 ("y"), s=w251, f=450.0) -> (s? t:f=w249:dbl)
                n87 = Divide(x=w258, y=w249) -> (x/y=w261:dbl)
                n88 = Divide(x=w244, y=50.0) -> (x/y=w254:dbl)
                n89 = Multiply(x=w261, y=16384.0) -> (x*y=w259:dbl)
                n90 = Multiply(x=w254, y=16384.0) -> (x*y=w256:dbl)
                n91 = Bundle By Name(cluster=T5 {"AO"=enum."Vout Variac", "Value"=0.0} ("Cluster SET AO"), "Value"=w259) -> (w263:T5)
                n92 = Bundle By Name(cluster=T5 {"AO"=enum."Vout Freq", "Value"=0.0} ("Cluster SET AO"), "Value"=w256) -> (w253:T5)
                n93 = Build Array(w263, w253) -> (w264:T5[])
                n94 = call "SET AO.vi"("Cluster SET AO"=w264) -> ()  [unwired: 10 in, 1 out]
              }
              frame True {
                w268 = 360.0 ("upper limit")
                w266 = 10.0 ("upper limit")
                n95 = In Range and Coerce(upper limit=w268, x=w271, lower limit=0.0) -> (coerced(x)=w269:dbl)  [unwired: 1 out]
                n96 = Divide(x=w269, y=w268) -> (x/y=w267:dbl)
                n97 = Multiply(x=w267, y=w266) -> (x*y=w265:dbl)
                n98 = In Range and Coerce(upper limit=w266, x=w265, lower limit=0.0) -> (coerced(x)=w272:dbl)  [unwired: 1 out]
                n99 = Bundle By Name(cluster=T5 {"AO"=enum."*V eccitazion", "Value"=0.0} ("Cluster SET AO"), "Value"=w272) -> (w275:T5)
                n100 = Build Array(w275) -> (w276:T5[])
                n101 = call "SET AO.vi"("Cluster SET AO"=w276) -> ()  [unwired: 10 in, 1 out]
              }
            }
          }
        }
        n102 = global write "tensione simulata.vi" "frequenza"(w148) -> ()
        n103 = Select(t=w176, s=w198, f=w177) -> (s? t:f=w200:string)
        n104 = Select(t=w178, s=w198, f=w179) -> (s? t:f=w199:string)
        n105 = property class="DigNum (strict)"(reference=w202, "Caption.Text"=w200) -> ()  [unwired: 1 in, 2 out]
        n106 = property class="DigNum (strict)"(reference=w201, "Caption.Text"=w199) -> ()  [unwired: 1 in, 2 out]
        n107 = local read "Stato Rampe"() -> (w217:T1)
        n108 = Bundle By Name(cluster=w217, "Fine rampa HZ"=w216, "Fine rampa V"=w215, "Tensione stabilizzata"=w214, "Fine rampa C"=w164, "Coppia stabilizzata"=w163, "Rampa Hz"=w148, "Rampa V"=w188, "Rampa C"=w162, "Trampa F(s)"=w210, "Trampa V(s)"=w211, "Trampa C(s)"=w161) -> (w212:T1)
        "Stato Rampe" <- w212
        n109 = global write "tensione simulata.vi" "tensione simulata"(w188) -> ()
        n110 = property class="Clust (strict)"(reference=w213, "Value"=w212) -> ()  [unwired: 1 in, 2 out]
        "Coppia letta" <- w157
      }
      frame "Aggiorna parametri rampe" {
        n111 = Variant To Data(type=T2 {"Frequenza"={"Tempo rampa (s)"=0.0, "Tempo stabiliz (s)"=0.0}, "Tensione"={"Tempo rampa (s)"=0.0, "Tempo stabiliz rampa(s)"=0.0, "Compensaz attiva?"=TRUE, "Precisione"=1.0, "Delta compensazione max"=30.0, "Time attesa stabiliz comp (s)"=5.0}, "Coppia"={"Tempo rampa (s)"=0.0, "Tempo stabiliz rampa(s)"=0.0, "Compensaz attiva?"=TRUE, "Precisione"=1.0, "Delta compensazione max"=30.0, "Time attesa stabiliz comp (s)"=5.0}} ("Parametri rampe e comp"), Variant=w287) -> (data=w278:T2)  [unwired: 1 in, 1 out]
        "stato Parametri rampe e comp" <- w278
        n112 = Unbundle By Name(w278) -> ("Coppia"=w285:T14, "Tensione"=w284:T14, "Frequenza"=w283:T15)
        n113 = property class="Clust (strict)"(reference=w279, "Value"=w278) -> ()  [unwired: 1 in, 2 out]
      }
      frame "Set V [V]" {
        n114 = Variant To Data(type=0.0 ("OUT"), Variant=w313) -> (data=w295:dbl)  [unwired: 1 in, 1 out]
        n115 = In Range and Coerce(upper limit=450.0, x=w295, lower limit=0.0) -> (coerced(x)=w297:dbl)  [unwired: 1 out]
        n116 = Not Equal To 0?(x=w295) -> (x != 0?=w294:bool)
        n117 = case shown="True" w294 {
          tunnel: w300 -> [_ w318]
          tunnel: w297 -> [_ w317]
          frame False {
          }
          frame True {
            n118 = property class="Clust (strict)"(reference=w318) -> (reference out=w315:refnum<vi>, "Value"=w316:cluster{"TENSIONE":dbl, "FREQUENZA":dbl})  [unwired: 1 in, 1 out]
            n119 = Bundle By Name(cluster=w316, "TENSIONE"=w317) -> (w314:cluster{"TENSIONE":dbl, "FREQUENZA":dbl})
            n120 = property class="Clust (strict)"(reference=w315, "Value"=w314) -> ()  [unwired: 1 in, 2 out]
          }
        }
      }
      frame "Set F [Hz]" {
        n121 = Variant To Data(type=0.0 ("OUT"), Variant=w337) -> (data=w323:dbl)  [unwired: 1 in, 1 out]
        n122 = In Range and Coerce(upper limit=100.0, x=w323, lower limit=0.0) -> (coerced(x)=w320:dbl)  [unwired: 1 out]
        n123 = Not Equal To 0?(x=w320) -> (x != 0?=w319:bool)
        n124 = case shown="False" w319 {
          tunnel: w325 -> [_ w343]
          tunnel: w320 -> [_ w342]
          frame False {
          }
          frame True {
            n125 = property class="Clust (strict)"(reference=w343) -> (reference out=w340:refnum<vi>, "Value"=w341:cluster{"TENSIONE":dbl, "FREQUENZA":dbl})  [unwired: 1 in, 1 out]
            n126 = Bundle By Name(cluster=w341, "FREQUENZA"=w342) -> (w339:cluster{"TENSIONE":dbl, "FREQUENZA":dbl})
            n127 = property class="Clust (strict)"(reference=w340, "Value"=w339) -> ()  [unwired: 1 in, 2 out]
          }
        }
      }
      frame "Set C [Nm]" {
        n128 = Variant To Data(type=0.0 ("OUT"), Variant=w361) -> (data=w347:dbl)  [unwired: 1 in, 1 out]
        n129 = In Range and Coerce(upper limit=50.0, x=w347, lower limit=0.0) -> (coerced(x)=w344:dbl)  [unwired: 1 out]
        n130 = property class="DigNum (strict)"(reference=w345, "Value"=w344) -> ()  [unwired: 1 in, 2 out]
      }
      frame "Exit" {
        n131 = property on="exit" class="Bool (strict)"("Val(Sgnl)"=TRUE ("Value (Signaling)")) -> ()  [unwired: 2 in, 2 out]
      }
    }
    n132 = Wait Until Next ms Multiple(millisecond multiple=w79) -> ()  [unwired: 1 out]
  }
  "error out" <- w7
  n133 = disable-structure shown="Disabled" {
    frame Disabled {
      n134 = call "calcolo compensazione C.vi"("P imp"="P imp", "P resa letta"="P resa letta", "RPM nom"="RPM nom", "RPM"="RPM", "precisione kw"="precisione kw") -> ()  [unwired: 9 in, 2 out]
    }
    frame Enabled {
    }
  }
